vi "hl_liberty_test.vi"   [LabVIEW 2014]
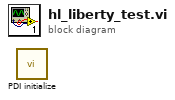
[diagram p0: block diagram]
diagram:
  n1 = call "PDI initialize.vi"() -> ()  [unwired: 5 in, 3 out]
